vi "UHR-Fleezers Control (host) -TL FB Corrected Ronen semipassive - stepping.vi"(0 "Tab Control":T5(tab)=enum."Trap Control (RF)") -> ()   [LabVIEW 2013] (continued)
                    n948 = Wait (ms)(milliseconds to wait=u32 500) -> ()  [unwired: 1 out]
                  }
                  frame #4 {
                    n949 = call "Write to pump.vi"("string"="start", "VISA resource name"=w1515) -> ()  [unwired: 1 out]
                  }
                }
              }
            }
          }
          frame Enabled {
            n950 = call "hamilton_controller.vi"("Open?"=w1517, "valve"=enum16{"A", "B", "C", "D", "ALL"}."A", "action"=T21."MOVE VALVE") -> ()  [unwired: 8 in, 1 out]
          }
        }
      }
      event "Inject Valve B": Value Change {
        n951 = event-data() -> ()  [unwired: 7 out]
        n952 = disable-structure shown="Enabled" {
          disable-tunnel: "Inject Valve B" -> [w1521 w1541]
          frame Disabled {
            n953 = local read "Pump write delay (ms)"() -> (w1523:dbl)
            n954 = flat-sequence {
              tunnel: w1522 -> [w1536]
              tunnel: w1523 -> [w1532]
              tunnel: w1521 -> [_]
              tunnel: w1523 -> [w1538]
              tunnel: w1522 -> [w1539]
              frame #0 {
                n955 = local read "All Pump Parameters"() -> (w1531:T6)
                n956 = Multiply(x=60.0, y="Flush Center Ch Rate (ul/m)") -> (x*y=w1528:dbl)
                n957 = Unbundle By Name(w1531) -> ("Pump 2"=w1537:T33)
                n958 = call "Set pump parameters.vi"("Pump write delay (ms)"=w1532, "Volume (uL)"="Flush Center Ch Volume (uL)", "Rate (uL/h)"=w1528, "Units"=3.0, "Pump #"=2.0, "Pump Parameters In"=w1537, "VISA resource name"=w1536) -> ("Pump Parameters Out"=w1530:T33)  [unwired: 3 in]
                n959 = Bundle By Name(cluster=w1531, "Pump 2"=w1530) -> (w1529:T6)
                n960 = local write "All Pump Parameters"(w1529) -> ()
                n961 = Add(x="Flush Center Ch Volume (uL)", y="Total Volume\nFlushed (uL)") -> (x+y=w1525:dbl)
                n962 = local write "Total Volume\nFlushed (uL)"(w1525) -> ()
              }
              frame #1 {
                n963 = Wait (ms)(milliseconds to wait=w1538) -> ()  [unwired: 1 out]
              }
              frame #2 {
                n964 = call "Write to pump.vi"("string"="start", "VISA resource name"=w1539) -> ()  [unwired: 1 out]
              }
            }
            n965 = local read "Chemyx Syringe Pump Serial Port"() -> (w1522:refnum<visa-resource-name>)
          }
          frame Enabled {
            n966 = call "hamilton_controller.vi"("Open?"=w1541, "valve"=enum16{"A", "B", "C", "D", "ALL"}."B", "action"=T21."MOVE VALVE") -> ()  [unwired: 8 in, 1 out]
          }
        }
      }
      event "Inject Bottom": Value Change {
        n967 = event-data() -> ()  [unwired: 7 out]
        n968 = call "hamilton_controller.vi"("Open?"="Inject Bottom", "valve"=enum16{"A", "B", "C", "D", "ALL"}."C", "action"=T21."MOVE VALVE") -> ()  [unwired: 8 in, 1 out]
      }
      event "Shunt:": Value Change {
        n969 = event-data() -> ()  [unwired: 7 out]
        n970 = call "hamilton_controller.vi"("Open?"="Shunt:", "valve"=enum16{"A", "B", "C", "D", "ALL"}."D", "action"=T21."MOVE VALVE") -> ()  [unwired: 8 in, 1 out]
      }
      event "Flip Green Filter": Value Change {
        n971 = event-data() -> ()  [unwired: 7 out]
        n972 = local write "Flip Green Filter"("Flip Green Filter") -> ()
        n973 = flat-sequence {
          tunnel: w1557 -> [w1562]
          tunnel: w1556 -> [w1561]
          tunnel: [w1559] -> w1554
          tunnel: [w1558] -> w1553
          tunnel: [w1564] -> w1552
          tunnel: w1554 -> [w1564]
          tunnel: [w1563] -> w1551
          tunnel: w1553 -> [w1563]
          tunnel: w1552 -> [w1568]
          tunnel: w1551 -> [w1567]
          tunnel: [w1566] -> w1555
          frame #0 {
            n974 = xnode "Read/Write Control"("FPGA VI Reference In"=w1562, "error in"=w1561, "Green Filter Flipper"=TRUE) -> ("FPGA VI Reference Out"=w1559:T20, "error out"=w1558:errorcluster)
          }
          frame #1 {
            n975 = Wait (ms)(milliseconds to wait=u32 100) -> ()  [unwired: 1 out]
          }
          frame #2 {
            n976 = xnode "Read/Write Control"("FPGA VI Reference In"=w1568, "error in"=w1567, "Green Filter Flipper"=FALSE) -> ("error out"=w1566:errorcluster)  [unwired: 1 out]
          }
        }
      }
      event "Pump 1 contents", "Pump 3 contents": Value Change {
        n977 = event-data() -> ()  [unwired: 7 out]
        n978 = local read "Pump 1 contents"() -> (→"Pump 1 cont disp":string)
        n979 = local read "Pump 3 contents"() -> (→"Pump 3 cont disp":string)
      }
      event "Reset Trap Pos. FB": Value Change {
        n980 = event-data() -> ()  [unwired: 7 out]
        n981 = xnode "Read/Write Control"("FPGA VI Reference In"=w1574, "error in"=w1573, "Trap Pos. FB Reset"="Reset Trap Pos. FB") -> ()  [unwired: 2 out]
      }
      event "Trap Pos. FB ON": Value Change {
        n982 = event-data() -> ()  [unwired: 7 out]
        n983 = xnode "Read/Write Control"("FPGA VI Reference In"=w1589, "error in"=w1588) -> ("FPGA VI Reference Out"=w1586:T20, "BD1 Frequency Out 1"=w1583:u64)  [unwired: 1 out]
        n984 = To Double Precision Float(number=w1583) -> (double precision float=w1582:dbl)
        n985 = Multiply(x=49125000.0, y=6.0) -> (x*y=w1581:dbl)
        n986 = Multiply(x=w1582, y=w1581) -> (x*y=w1579:dbl)
        n987 = Scale By Power Of 2(n=-48, x=w1579) -> (x*2^n=w1578:dbl)
        n988 = Divide(x=w1578, y=1000000.0) -> (x/y=w1575:dbl)
        n989 = flat-sequence {
          tunnel: [w1592] -> w1587
          tunnel: w1586 -> [w1593]
          tunnel: w1583 -> [w1591]
          tunnel: "Trap Pos. FB ON" -> [w1590]
          tunnel: "Trap Pos. FB ON" -> [w1599]
          tunnel: w1587 -> [w1598]
          tunnel: "Trap Pos. FB ON" -> [w1601]
          tunnel: w1575 -> [w1600]
          frame #0 {
            n990 = case shown="False" w1590 {
              tunnel: w1593 -> [w1596 w1597]
              tunnel: [w1595 w1597] -> w1592
              tunnel: w1591 -> [w1594 _]
              frame False {
                n991 = xnode "Read/Write Control"("FPGA VI Reference In"=w1596, "BD 1 Frequency 1"=w1594) -> ("FPGA VI Reference Out"=w1595:T20)  [unwired: 1 in, 1 out]
              }
              frame True {
              }
            }
          }
          frame #1 {
            n992 = xnode "Read/Write Control"("FPGA VI Reference In"=w1598, "Force feedback"=w1599) -> ()  [unwired: 1 in, 2 out]
          }
          frame #2 {
            n993 = case shown="False" w1601 {
              tunnel: w1600 -> [w1603 _]
              frame False {
                n994 = Subtract(x=90.0, y=w1603) -> (x-y=w1602:dbl)
                n995 = property on="Trap Delta (MHz)" class="DigNum (strict)"("Val(Sgnl)"=w1602) -> ()  [unwired: 2 in, 2 out]
              }
              frame True {
              }
            }
          }
        }
      }
      event "Diff. FB.", "Trap Pos. FB Gains", "Trap Pos. FB Mult Factor", "Trap Pos. FB Offset Factor", "Trap Pos FB Negate Action", "Trap Pos FB Monitor\nT1 or T2", "Negate Diff?": Value Change {
        n996 = event-data() -> ()  [unwired: 7 out]
        n997 = xnode "Read/Write Control"("FPGA VI Reference In"=w1615, "error in"=w1614, "Trap Pos. FB Range"="Trap Pos. FB Range", "Trap Pos. FB Gains"="Trap Pos. FB Gains", "Trap Pos. FB Mult Factor"="Trap Pos. FB Mult Factor", "Trap Pos. FB Offset Factor"="Trap Pos. FB Offset Factor", "Trap Pos FB Negate Action"="Trap Pos FB Negate Action", "Trap Pos FB Monitor T1 or T2"="Trap Pos FB Monitor\nT1 or T2", "AI1 X Scale"="Trap Pos. AI1 X Pre-scale", "Negate Diff?"="Negate Diff?", "Diff FB Measurement?"="Diff. FB.") -> ()  [unwired: 2 out]
      }
      event "Trap Pos FB SP": Value Change {
        n998 = event-data() -> ()  [unwired: 7 out]
        n999 = xnode "Read/Write Control"("FPGA VI Reference In"=w1618, "error in"=w1617, "Trap Pos. FB SP"="Trap Pos FB SP") -> ()  [unwired: 2 out]
      }
      event "Simulate stepping": Value Change {
        n1000 = event-data() -> ()  [unwired: 7 out]
        n1001 = flat-sequence {
          tunnel: w1620 -> [w1623]
          tunnel: [w1622] -> _
          tunnel: w1619 -> [w1621]
          frame #0 {
            n1002 = while {
              tunnel: w1623 -> [w1651]
              tunnel: [w1650] -> w1622 mode=indexing
              tunnel: w1621 -> [w1649]
              i -> [w1635]
              stop <- w1632 stop-if-true
              w1625 = 1000.0
              n1003 = Divide(x="Backtrack probability", y=100) -> (x/y=w1659:dbl)
              n1004 = Random Number (0-1)() -> (number: 0 to 1=w1660:dbl)
              n1005 = Greater?(x=w1660, y=w1659) -> (0:w1658:bool)
              n1006 = Select(t=1, s=w1658, f=-1) -> (s? t:f=w1655:i32)
              n1007 = local read "BD 1 Frequency 2 (MHz)"() -> (w1630:dbl)
              n1008 = Multiply(x=w1655, y="Step size (nm)") -> (x*y=w1653:dbl)
              "Step taken" <- w1653
              n1009 = Divide(x=w1653, y=168.33) -> (x/y=w1628:dbl)
              n1010 = local read "BD 1 Frequency 1 (MHz)"() -> (w1629:dbl)
              n1011 = local read "X RF Frequency Limits (MHz)"() -> (w1648:T17)
              n1012 = local read "Y RF Frequency Limits (MHz)"() -> (w1647:T17)
              n1013 = Subtract(x=w1629, y=w1628) -> (x-y=w1627:dbl)
              n1014 = local write "BD 1 Frequency 1 (MHz)"(w1627) -> ()
              n1015 = local read "BD 2 Frequency 1 (MHz)"() -> (w1645:dbl)
              n1016 = local read "BD 2 Frequency 2 (MHz)"() -> (w1646:dbl)
              n1017 = call "set RF board frequency - interlace.vi"("Board 2 Frequency Limits"=w1647, "Board 1 Frequency Limits"=w1648, "error in"=w1651, "FPGA VI Reference In"=w1649, "Board 2 Frequency 2 (MHz)"=w1646, "Board 2 Frequency 1 (MHz)"=w1645, "Board 1 Frequency 2 (MHz)"=w1630, "Board 1 Frequency 1  (MHz)"=w1627) -> ("error out"=w1650:errorcluster)  [unwired: 2 in, 1 out]
              n1018 = Subtract(x=w1630, y=w1627) -> (x-y=w1644:dbl)
              n1019 = Subtract(x=w1646, y=w1645) -> (x-y=w1643:dbl)
              n1020 = Square(x=w1643) -> (x^2=w1641:dbl)
              n1021 = Square(x=w1644) -> (x^2=w1642:dbl)
              n1022 = Add(x=w1642, y=w1641) -> (x+y=w1640:dbl)
              n1023 = Square Root(x=w1640) -> (sqrt(x)=w1631:dbl)
              n1024 = local write "Trap Delta (MHz)"(w1631) -> ()
              n1025 = property on="Initial delta (MHz)" class="DigNum (strict)"("Val(Sgnl)"=w1631) -> ()  [unwired: 2 in, 2 out]
              n1026 = Multiply(x="Mean dwell time (s)", y=w1625) -> (x*y=w1637:dbl)
              n1027 = case shown="\"Gamma2\"" "Distribution" {
                tunnel: w1637 -> [w1664 w1668 w1671]
                tunnel: [w1664 w1665 w1672] -> w1626
                frame "uniform", Default {
                }
                frame "Exponential" {
                  n1028 = call-poly <vilib>:"Continuous Random.vi"("b"=w1668, "samples"=1) -> ("exp random data"=w1666:dbl[])  [unwired: 8 in, 1 out]
                  n1029 = Index Array(array=w1666) -> (element=w1665:dbl)  [unwired: 1 in]
                }
                frame "Gamma2" {
                  w1669 = 2.0
                  # "Note: the shape and scale\nparameters of the gamma\nare inverted because LabView..."
                  n1030 = Divide(x=w1671, y=w1669) -> (x/y=w1670:dbl)
                  n1031 = call-poly <vilib>:"Continuous Random.vi"("c"=w1670, "b"=w1669, "samples"=1) -> ("gamma random numbers"=w1673:dbl[])  [unwired: 7 in, 1 out]
                  n1032 = Index Array(array=w1673) -> (element=w1672:dbl)  [unwired: 1 in]
                }
              }
              n1033 = Divide(x=w1626, y=w1625) -> (x/y=→"Step duration":dbl)
              n1034 = To Unsigned Long Integer(number=w1626) -> (unsigned 32bit integer=w1638:u32)
              n1035 = Add(x=w1635, y=1) -> (x+y=w1634:i32)
              n1036 = Wait (ms)(milliseconds to wait=w1638) -> ()  [unwired: 1 out]
              n1037 = Equal?(x=w1634, y="Number of steps") -> (x = y?=w1632:bool)
            }
          }
          frame #1 {
            n1038 = local write "Simulate stepping"(FALSE) -> ()
          }
        }
      }
      event "Set SP to Reading": Value Change {
        n1039 = event-data() -> ()  [unwired: 7 out]
        n1040 = local read "Trap Pos FB Monitor\nT1 or T2"() -> (w1683:bool)
        n1041 = local read "Trap X AI1 (DMA)"() -> (w1686:T13)
        n1042 = local read "Trap X (AI1)"() -> (w1689:T1)
        n1043 = Unbundle By Name(w1689) -> ("Trap 1"=w1688:fxp<+/-,16,1>, "Trap 2"=w1687:fxp<+/-,16,1>)
        n1044 = Unbundle By Name(w1686) -> ("Set 1"=w1685:fxp<+/-,16,1>, "Set 2"=w1684:fxp<+/-,16,1>)
        n1045 = Select(t=w1688, s=w1683, f=w1687) -> (s? t:f=w1682:fxp<+/-,16,1>)
        n1046 = Select(t=w1685, s=w1683, f=w1684) -> (s? t:f=w1681:fxp<+/-,16,1>)
        n1047 = Not(x="Set SP Using...") -> (.not. x?=w1676:bool)
        n1048 = Select(t=w1682, s=w1676, f=w1681) -> (s? t:f=w1677:fxp<+/-,16,1>)
        n1049 = xnode "Read/Write Control"("FPGA VI Reference In"=w1679, "error in"=w1678, "Trap Pos. FB SP"=w1677) -> ()  [unwired: 2 out]
        n1050 = local write "Trap Pos FB SP"(w1677) -> ()
      }
      event "Trap Pos. FB Out Scale 2^n": Value Change {
        n1051 = event-data() -> ()  [unwired: 7 out]
        n1052 = Scale By Power Of 2(n="Trap Pos. FB Out Scale 2^n", x=ext 1.0) -> (x*2^n=w1691:ext)
        n1053 = property on="Trap Pos. FB Mult Factor" class="DigNum (strict)"("Val(Sgnl)"=w1691) -> ()  [unwired: 2 in, 2 out]
      }
      event "Trap Pos FB Int Count": Value Change {
        n1054 = event-data() -> ()  [unwired: 7 out]
        n1055 = xnode "Read/Write Control"("FPGA VI Reference In"=w1696, "error in"=w1695, "Trap Pos FB Int Count"="Trap Pos FB Int Count") -> ()  [unwired: 2 out]
      }
      event "Target Force (pN)", "Setpoint offset\nCorrection values": Value Change {
        n1056 = event-data() -> ()  [unwired: 7 out]
        n1057 = local read "B factor"() -> (w1729:dbl)
        n1058 = To Fixed-Point(number=w1729) -> (fixed-point=w1728:fxp<+/-,16,16>)  [unwired: 1 in]
        n1059 = xnode "Read/Write Control"("FPGA VI Reference In"=w1730, "B factor"=w1728) -> ("BD1 Frequency Out 1"=w1719:u64)  [unwired: 1 in, 2 out]
        n1060 = local read "BD 1 Frequency 2 (MHz)"() -> (w1718:dbl)
        n1061 = local read "Target Force (pN)"() -> (w1704:dbl)
        n1062 = To Double Precision Float(number=w1719) -> (double precision float=w1725:dbl)
        n1063 = Multiply(x=49125000.0, y=6.0) -> (x*y=w1724:dbl)
        n1064 = Multiply(x=w1725, y=w1724) -> (x*y=w1722:dbl)
        n1065 = Scale By Power Of 2(n=-48, x=w1722) -> (x*2^n=w1721:dbl)
        n1066 = Divide(x=w1721, y=1000000.0) -> (x/y=w1717:dbl)
        n1067 = Subtract(x=w1718, y=w1717) -> (x-y=w1716:dbl)
        n1068 = local read "T1 kappa_x (pN/nm)"() -> (w1705:dbl)
        n1069 = local read "T1 alpha_x (nm/V)"() -> (w1706:dbl)
        n1070 = local read "Negate offset difference"() -> (w1707:bool)
        n1071 = local read "Offset file step size"() -> (w1715:dbl)
        n1072 = Multiply(x=w1704, y=2.0) -> (x*y=w1702:dbl)
        n1073 = local read "Setpoint offset\nCorrection values"() -> (w1712:dbl[])
        n1074 = Divide(x=w1716, y=w1715) -> (x/y=w1714:dbl)
        n1075 = Select(t=-1, s=w1707, f=1) -> (s? t:f=w1708:i32)
        n1076 = To Long Integer(number=w1714) -> (32bit integer=w1713:i32)
        n1077 = Multiply(x=w1706, y=w1705) -> (x*y=w1701:dbl)
        n1078 = Divide(x=w1702, y=w1701) -> (x/y=w1700:dbl)
        n1079 = Index Array(array=w1712, index=w1713) -> (element=w1711:dbl)
        n1080 = Multiply(x=w1708, y=w1711) -> (x*y=w1699:dbl)
        n1081 = Add(x=w1700, y=w1699) -> (x+y=w1698:dbl)
        n1082 = To Fixed-Point(number=w1698) -> (fixed-point=w1697:fxp<+/-,16,1>)  [unwired: 1 in]
        n1083 = property on="Trap Pos FB SP" class="DigNum (strict)"("Val(Sgnl)"=w1697) -> ()  [unwired: 2 in, 2 out]
      }
      event "Read setpoint correction\nfile": Value Change {
        n1084 = event-data() -> ()  [unwired: 7 out]
        n1085 = local write "Read setpoint correction\nfile"(FALSE) -> ()
        n1086 = Open/Create/Replace File(file path (use dialog)="Setpoint correction\noffset file", operation (0:open)=T24."open", access (0:read/write)=enum16{"read/write", "read-only", "write-only"}."read-only") -> (refnum out=w1755:refnum<file>)  [unwired: 1 in, 4 out]
        n1087 = Deny Access(7:w1755) -> (3:w1753:refnum<file>)  [unwired: 1 in, 2 out]
        n1088 = Read from Binary File(5:0.0, 9:T30."big-endian, network order" ("byte order (0:big-endian, network order)"), 10:-1 ("count (1)"), 11:w1753) -> (2:w1746:dbl[], 3:w1752:refnum<file>)  [unwired: 1 in, 3 out]
        n1089 = Close File(refnum=w1752) -> ()  [unwired: 1 in, 2 out]
        n1090 = Index Array(array=w1746, index=0) -> (element=w1742:dbl)
        n1091 = local write "Offset file step size"(w1742) -> ()
        n1092 = Array Subset(array=w1746, index=3) -> (w1745:dbl[])  [unwired: 1 in]
        n1093 = local read "T1 kappa_x (pN/nm)"() -> (w1740:dbl)
        n1094 = local read "T1 alpha_x (nm/V)"() -> (w1741:dbl)
        n1095 = local read "T2 alpha_x (nm/V)"() -> (w1739:dbl)
        n1096 = local read "T2 kappa_x (pN/nm)"() -> (w1738:dbl)
        n1097 = Decimate 1D Array(w1745) -> (w1733:dbl[], w1734:dbl[])  [unwired: 1 out]
        n1098 = local read "Offset Values"() -> (w1744:T14)
        n1099 = Multiply(x=w1741, y=w1740) -> (x*y=w1736:dbl)
        n1100 = Multiply(x=w1739, y=w1738) -> (x*y=w1737:dbl)
        n1101 = Bundle By Name(cluster=w1744, "Trap 1X offset"=w1733, "Trap 2X offset"=w1734) -> (w1743:T14)
        n1102 = Divide(x=w1737, y=w1736) -> (x/y=w1735:dbl)
        n1103 = property on="B factor" class="DigNum (strict)"("Val(Sgnl)"=w1735) -> ()  [unwired: 2 in, 2 out]
        n1104 = Multiply(x=w1734, y=w1735) -> (x*y=w1732:dbl[])
        n1105 = local write "Offset Values"(w1743) -> ()
        n1106 = Subtract(x=w1733, y=w1732) -> (x-y=w1731:dbl[])
        n1107 = property on="Setpoint offset\nCorrection values" class="Arr (strict)"("Val(Sgnl)"=w1731) -> ()  [unwired: 2 in, 2 out]
      }
      event "MCL Tracking": Value Change {
        n1108 = event-data() -> ()  [unwired: 7 out]
        n1109 = case shown="True" "MCL Tracking" {
          frame False {
            n1110 = local read "Current MCL (V)"() -> (w1760:dbl)
            n1111 = local write "AO2"(w1760) -> ()
          }
          frame True {
            n1112 = local read "BD 1 Frequency 1 (MHz)"() -> (→"Zero T1 position":dbl)
            n1113 = local read "AO2"() -> (→"Zero MCL x position":dbl)
          }
        }
      }
    }
    "error out 2" <- w754
    n1114 = node-c288() -> ()  [unwired: 1 in, 1 out]
  }
  n1115 = timed-loop "Run Scripts, including: stage motion" {
    timing: w89 -> [_]
    timing-out: [_] -> w88
    tunnel: w44 -> [_]
    stop <- w1764 stop-if-true
    n1116 = node-c288() -> ()  [unwired: 1 in, 1 out]
    n1117 = event shown="[2] \"Cal/Data Acq. Spot\": Value Change" {
      selector: _ -> [_ _ _ _ _ _ _ _ _ _ _ _]
      dyn-events: _ -> [_ _ _ _ _ _ _ _ _ _ _ _]
      timeout: 50 -> [_ _ _ _ _ _ _ _ _ _ _ _]
      tunnel: ["Move Cap. 1 (DNA Top)" _ "Cal/Data Acq. Spot" "Dump Beads" "Dip for Protein" _ "Got ADig bead" "Got DNA bead" "Take Stepping Data" _ "Take Detection Laser\nImage" _] -> _
      tunnel: [_ _ _ _ _ _ _ _ _ _ _ w1972] -> w1764
      event "Move Cap. 1 (DNA Top)": Value Change {
        n1118 = event-data() -> ()  [unwired: 1 in, 5 out]
        n1119 = local write "Move Cap. 1 (DNA Top)"(FALSE ("Move Cap. 1 (DNA Right)")) -> ()
        n1120 = flat-sequence {
          tunnel: "Cap 1 Samp Flow ON" -> [w1770]
          frame #0 {
            n1121 = local write "Stage Moving"(FALSE ("Stage Moving")) -> ()
            n1122 = case "stop flow" shown="True" w1770 {
              frame False {
              }
              frame True {
                n1123 = call "hamilton_controller.vi"("Open?"=FALSE, "valve"=enum16{"A", "B", "C", "D", "ALL"}."C", "action"=T21."MOVE VALVE") -> ()  [unwired: 8 in, 1 out]
              }
            }
            n1124 = case shown="True" TRUE {
              tunnel: "Cap 1 T ON" -> [w1779 w1780]
              frame False {
                n1125 = property on="Trap 1 (ON/OFF)" class="Bool (strict)"("Val(Sgnl)"=w1779) -> ()  [unwired: 2 in, 2 out]
              }
              frame True {
                n1126 = property on="Trap 2 (ON/OFF)" class="Bool (strict)"("Val(Sgnl)"=w1780) -> ()  [unwired: 2 in, 2 out]
              }
            }
            n1127 = call <vilib>:"Beep.vi"() -> ()  [unwired: 3 in, 9 out]
            n1128 = case shown="True" "Cap 1 Flow ON" {
              frame False {
              }
              frame True {
                n1129 = property on="Main:" class="Bool (strict)"("Val(Sgnl)"=TRUE ("Value (Signaling)")) -> ()  [unwired: 2 in, 2 out]
              }
            }
          }
        }
      }
      event Timeout {
        n1130 = event-data() -> ()  [unwired: 1 in, 2 out]
      }
      event "Cal/Data Acq. Spot": Value Change {
        # "wait for calibration file\nto be written"
        # "signal save cal true\nthis tells the data \nacquisition loop to\nstart sending the data\nto a calibration file"
        # "separate traps to\nthe desired trap delta"
        # "move stage to data acquisition spot"
        # "CHANGE FISH FOR TETHER BACK\nTO TRUE VALUE HERE."
        n1131 = event-data() -> ()  [unwired: 1 in, 5 out]
        n1132 = local write "Cal/Data Acq. Spot"(FALSE ("Cal/Data Acq. Spot")) -> ()
        n1133 = flat-sequence {
          tunnel: ["Cal @ (MHz)"] -> w1781
          tunnel: w1781 -> [w1791]
          tunnel: w1781 -> [w1812]
          frame #0 {
            n1134 = property on="Trap Delta (MHz)" class="DigNum (strict)"("Val(Sgnl)"="Cal @ (MHz)") -> ()  [unwired: 2 in, 2 out]
            n1135 = call <vilib>:"Beep.vi"() -> ()  [unwired: 3 in, 9 out]
          }
          frame #1 {
            n1136 = Wait (ms)(milliseconds to wait=u32 100) -> ()  [unwired: 1 out]
          }
          frame #2 {
            n1137 = property on="Save Calibration" class="Bool (strict)"("Val(Sgnl)"=TRUE ("Value (Signaling)")) -> ()  [unwired: 2 in, 2 out]
          }
          frame #3 {
            n1138 = Wait (ms)(milliseconds to wait=u32 4000) -> ()  [unwired: 1 out]
          }
          frame #4 {
            n1139 = while {
              stop <- w1788 stop-if-true
              n1140 = local read "Saving..."() -> (w1789:bool)
              n1141 = Wait (ms)(milliseconds to wait=u32 100) -> ()  [unwired: 1 out]
              n1142 = Not(x=w1789) -> (.not. x?=w1788:bool)
            }
          }
          frame #5 {
            n1143 = case shown="True" "W/ Offset 1" {
              tunnel: w1791 -> [_ w1793]
              frame False {
              }
              frame True {
                n1144 = stacked-sequence {
                  tunnel: w1793 -> [_ _ _ _ _ _ _ w1810]
                  frame #0 {
                    n1145 = Replace Array Subset(array=u32[] [0] ("Index Values"), new element="Offset 1 Set", index=0) -> (w1794:u32[])
                    n1146 = property on="Saved AOD Raster Scan Parameter Sets" class="Arr (strict)"("Index Values"=w1794) -> ()  [unwired: 2 in, 2 out]
                    n1147 = property on="Trap Delta (MHz)" class="DigNum (strict)"("Val(Sgnl)"="Offset 1 Start (MHz)") -> ()  [unwired: 2 in, 2 out]
                  }
                  frame #1 {
                    n1148 = Wait (ms)(milliseconds to wait=u32 200) -> ()  [unwired: 1 out]
                  }
                  frame #2 {
                    n1149 = property on="Load parameters" class="Bool (strict)"("Val(Sgnl)"=TRUE ("Value (Signaling)")) -> ()  [unwired: 2 in, 2 out]
                  }
                  frame #3 {
                    n1150 = Wait (ms)(milliseconds to wait=u32 200) -> ()  [unwired: 1 out]
                  }
                  frame #4 {
                    n1151 = property on="Trap Raster Scan" class="Bool (strict)"("Val(Sgnl)"=TRUE ("Value (Signaling)")) -> ()  [unwired: 2 in, 2 out]
                  }
                  frame #5 {
                    n1152 = Wait (ms)(milliseconds to wait=u32 2000) -> ()  [unwired: 1 out]
                  }
                  frame #6 {
                    n1153 = while {
                      stop <- w1807 stop-if-true
                      n1154 = local read "Raster Scanning..."() -> (w1809:bool)
                      n1155 = local read "Saving..."() -> (w1805:bool)
                      n1156 = Wait (ms)(milliseconds to wait=u32 100) -> ()  [unwired: 1 out]
                      n1157 = Not(x=w1805) -> (.not. x?=w1804:bool)
                      n1158 = Not(x=w1809) -> (.not. x?=w1806:bool)
                      n1159 = And(x=w1806, y=w1804) -> (x .and. y?=w1807:bool)
                    }
                  }
                  frame #7 {
                    n1160 = property on="Trap Delta (MHz)" class="DigNum (strict)"("Val(Sgnl)"=w1810) -> ()  [unwired: 2 in, 2 out]
                  }
                }
              }
            }
          }
          frame #6 {
            n1161 = local read "Save ave N"() -> (w1811:dbl)
            n1162 = case shown="True" "W/ Offset 2" {
              tunnel: w1812 -> [_ w1818]
              tunnel: w1811 -> [_ w1817]
              frame False {
                n1163 = Multiply(x="Cal read wait (s)", y=u32 1000 ("milliseconds to wait")) -> (x*y=w1815:u32)
                n1164 = Wait (ms)(milliseconds to wait=w1815) -> ()  [unwired: 1 out]
              }
              frame True {
                n1165 = stacked-sequence {
                  tunnel: w1818 -> [_ _ _ _ _ _ _ _ _ w1839 _ _]
                  tunnel: w1817 -> [_ _ _ _ _ _ _ _ _ w1837 _ _]
                  frame #0 {
                    n1166 = property on="Save ave N" class="DigNum (strict)"("Val(Sgnl)"=1.0 ("Value (Signaling)")) -> ()  [unwired: 2 in, 2 out]
                  }
                  frame #1 {
                    n1167 = Wait (ms)(milliseconds to wait=u32 500) -> ()  [unwired: 1 out]
                  }
                  frame #2 {
                    n1168 = property on="Trap Delta (MHz)" class="DigNum (strict)"("Val(Sgnl)"="Offset 2 Start (MHz)") -> ()  [unwired: 2 in, 2 out]
                    n1169 = Replace Array Subset(array=u32[] [0] ("Index Values"), new element="Offset 2 Set", index=0) -> (w1823:u32[])
                    n1170 = property on="Saved AOD Raster Scan Parameter Sets" class="Arr (strict)"("Index Values"=w1823) -> ()  [unwired: 2 in, 2 out]
                  }
                  frame #3 {
                    n1171 = Wait (ms)(milliseconds to wait=u32 500) -> ()  [unwired: 1 out]
                  }
                  frame #4 {
                    n1172 = property on="Load parameters" class="Bool (strict)"("Val(Sgnl)"=TRUE ("Value (Signaling)")) -> ()  [unwired: 2 in, 2 out]
                  }
                  frame #5 {
                    n1173 = Wait (ms)(milliseconds to wait=u32 500) -> ()  [unwired: 1 out]
                  }
                  frame #6 {
                    n1174 = property on="Trap Raster Scan" class="Bool (strict)"("Val(Sgnl)"=TRUE ("Value (Signaling)")) -> ()  [unwired: 2 in, 2 out]
                  }
                  frame #7 {
                    n1175 = Wait (ms)(milliseconds to wait=u32 2000) -> ()  [unwired: 1 out]
                  }
                  frame #8 {
                    n1176 = while {
                      stop <- w1832 stop-if-true
                      n1177 = local read "Raster Scanning..."() -> (w1835:bool)
                      n1178 = local read "Saving..."() -> (w1833:bool)
                      n1179 = Wait (ms)(milliseconds to wait=u32 100) -> ()  [unwired: 1 out]
                      n1180 = Not(x=w1833) -> (.not. x?=w1831:bool)
                      n1181 = Not(x=w1835) -> (.not. x?=w1834:bool)
                      n1182 = And(x=w1834, y=w1831) -> (x .and. y?=w1832:bool)
                    }
                  }
                  frame #9 {
                    n1183 = property on="Trap Delta (MHz)" class="DigNum (strict)"("Val(Sgnl)"=w1839) -> ()  [unwired: 2 in, 2 out]
                    n1184 = property on="Saved AOD Raster Scan Parameter Sets" class="Arr (strict)"("Index Values"=u32[] [0]) -> ()  [unwired: 2 in, 2 out]
                    n1185 = property on="Save ave N" class="DigNum (strict)"("Val(Sgnl)"=w1837) -> ()  [unwired: 2 in, 2 out]
                  }
                  frame #10 {
                    n1186 = Wait (ms)(milliseconds to wait=u32 500) -> ()  [unwired: 1 out]
                  }
                  frame #11 {
                    n1187 = property on="Load parameters" class="Bool (strict)"("Val(Sgnl)"=TRUE ("Value (Signaling)")) -> ()  [unwired: 2 in, 2 out]
                  }
                }
              }
            }
          }
          frame #7 {
            n1188 = property on="Read Cal" class="Bool (strict)"("Val(Sgnl)"=TRUE ("Value (Signaling)")) -> ()  [unwired: 2 in, 2 out]
          }
          frame #8 {
            n1189 = Wait (ms)(milliseconds to wait=u32 500) -> ()  [unwired: 1 out]
          }
          frame #9 {
            n1190 = property on="Fish for Tether" class="Bool (strict)"("Val(Sgnl)"=FALSE ("Value (Signaling)")) -> ()  [unwired: 2 in, 2 out]
          }
        }
      }
      event "Dump Beads": Value Change {
        # "SCRIPT TO REMOVE BOTH BEADS FROM THE TRAPS. TURNS ON LIGHT WHICH INDICATES THAT STAGE IS MOVING. THEN STOPS SAVING DATA. \nSETS Sample Channel Flow TO TRUE. STOPS INTERLACING GREEN FLUORESCENCE. TURNS OFF Tether INDICATOR BECAUSE WE ARE THROWING IT\nAWAY. SHUTS OFF TRAP POSITION FEEDBACK."
        n1191 = event-data() -> ()  [unwired: 1 in, 5 out]
        n1192 = flat-sequence {
          frame #0 {
            w1846 = FALSE ("Fl. Triggered...")
            w1847 = TRUE ("Stage Moving")
            n1193 = local read "Saving..."() -> (w1848:bool)
            n1194 = local write "Fl. Triggered..."(w1846) -> ()
            n1195 = local write "Stage Moving"(w1847) -> ()
            n1196 = local write "Tether"(w1846) -> ()
            n1197 = property on="Green Laser ON/Interlacing" class="Bool (strict)"("Val(Sgnl)"=w1846) -> ()  [unwired: 2 in, 2 out]
            n1198 = property on="Trap Pos. FB ON" class="Bool (strict)"("Val(Sgnl)"=w1846) -> ()  [unwired: 2 in, 2 out]
            n1199 = property on="Inject Bottom" class="Bool (strict)"("Val(Sgnl)"=w1847) -> ()  [unwired: 2 in, 2 out]
            n1200 = local write "Stop Saving"(w1848) -> ()
          }
          frame #1 {
            w1849 = FALSE ("Value (Signaling)")
            # "TURNS TRAPS OFF SO THAT\nBEADS REMAIN AT DUMP \nBEADS POSITION"
            n1201 = property on="Trap 1 (ON/OFF)" class="Bool (strict)"("Val(Sgnl)"=w1849) -> ()  [unwired: 2 in, 2 out]
            n1202 = property on="Trap 2 (ON/OFF)" class="Bool (strict)"("Val(Sgnl)"=w1849) -> ()  [unwired: 2 in, 2 out]
            n1203 = call <vilib>:"Beep.vi"() -> ()  [unwired: 3 in, 9 out]
          }
          frame #2 {
            n1204 = property on="Goto Bottom (F7)" class="Bool (strict)"("Val(Sgnl)"=TRUE ("Value (Signaling)")) -> ()  [unwired: 2 in, 2 out]
          }
          frame #3 {
            n1205 = Wait (ms)(milliseconds to wait=u32 8000) -> ()  [unwired: 1 out]
          }
          frame #4 {
            n1206 = property on="Trap Delta (MHz)" class="DigNum (strict)"("Val(Sgnl)"=20.0 ("Value (Signaling)")) -> ()  [unwired: 2 in, 2 out]
          }
          frame #5 {
            n1207 = property on="Trap 2 (ON/OFF)" class="Bool (strict)"("Val(Sgnl)"=TRUE ("Value (Signaling)")) -> ()  [unwired: 2 in, 2 out]
          }
          frame #6 {
            n1208 = property on="Inject Bottom" class="Bool (strict)"("Val(Sgnl)"=FALSE ("Value (Signaling)")) -> ()  [unwired: 2 in, 2 out]
          }
        }
      }
      event "Dip for Protein": Value Change {
        n1209 = event-data() -> ()  [unwired: 1 in, 5 out]
        n1210 = flat-sequence {
          frame #0 {
            n1211 = case shown="True" "Move Trap Before?" {
              frame False {
              }
              frame True {
                n1212 = property on="Trap Delta (MHz)" class="DigNum (strict)"("Val(Sgnl)"="Dip Trap Delta 1 (MHz)") -> ()  [unwired: 2 in, 2 out]
              }
            }
          }
          frame #1 {
            n1213 = Multiply(x="Duration (s)", y=1000.0) -> (x*y=w1858:dbl)
            n1214 = Wait (ms)(milliseconds to wait=w1858) -> ()  [unwired: 1 out]
          }
          frame #2 {
            n1215 = case shown="True" "Move Trap After?" {
              frame False {
              }
              frame True {
                n1216 = property on="Trap Delta (MHz)" class="DigNum (strict)"("Val(Sgnl)"="Dip Trap Delta 2 (MHz)") -> ()  [unwired: 2 in, 2 out]
              }
            }
          }
          frame #3 {
            n1217 = case shown="True" "Green ON After?" {
              frame False {
              }
              frame True {
                n1218 = property on="Green Laser ON/Interlacing" class="Bool (strict)"("Val(Sgnl)"=TRUE ("Value (Signaling)")) -> ()  [unwired: 2 in, 2 out]
              }
            }
          }
          frame #4 {
            n1219 = Wait (ms)(milliseconds to wait=u32 500) -> ()  [unwired: 1 out]
          }
          frame #5 {
            n1220 = case shown="True" "Save Data After?" {
              frame False {
              }
              frame True {
                n1221 = property on="Start Saving" class="Bool (strict)"("Val(Sgnl)"=TRUE ("Value (Signaling)")) -> ()  [unwired: 2 in, 2 out]
              }
            }
          }
        }
      }
      event "Profile": Value Change {
        n1222 = event-data() -> ()  [unwired: 1 in, 5 out]
        n1223 = flat-sequence {
          frame #0 {
            w1868 = 0.0 ("element")
            n1224 = Build Array(w1868, "Y change (mm)", w1868) -> ()  [unwired: 1 out]
          }
          frame #1 {
            # "stop saving"
            n1225 = local write "Stop Saving"(TRUE ("Stop Saving")) -> ()
            n1226 = local write "Stage Moving"(FALSE ("Stage Moving")) -> ()
          }
        }
      }
      event "Got ADig bead": Value Change {
        n1227 = event-data() -> ()  [unwired: 1 in, 5 out]
        n1228 = property on="Move Cap. 1 (DNA Top)" class="Bool (strict)"("Val(Sgnl)"=TRUE ("Value (Signaling)")) -> ()  [unwired: 2 in, 2 out]
        n1229 = property on="Inject Top:" class="Bool (strict)"("Val(Sgnl)"=FALSE ("Value (Signaling)")) -> ()  [unwired: 2 in, 2 out]
      }
      event "Got DNA bead": Value Change {
        n1230 = event-data() -> ()  [unwired: 1 in, 5 out]
        n1231 = property on="Cal/Data Acq. Spot" class="Bool (strict)"("Val(Sgnl)"=TRUE ("Value (Signaling)")) -> ()  [unwired: 2 in, 2 out]
        n1232 = property on="Main:" class="Bool (strict)"("Val(Sgnl)"=FALSE ("Value (Signaling)")) -> ()  [unwired: 2 in, 2 out]
      }
      event "Take Stepping Data": Value Change {
        n1233 = event-data() -> ()  [unwired: 1 in, 5 out]
        n1234 = local read "Save ave N"() -> (w1886:dbl)
        n1235 = flat-sequence {
          tunnel: w1886 -> [w1888]
          tunnel: [w1888] -> w1881
          tunnel: [w1890] -> w1882
          tunnel: w1881 -> [w1890]
          tunnel: [w1892] -> w1883
          tunnel: w1882 -> [w1892]
          tunnel: [w1895] -> w1884
          tunnel: w1883 -> [w1895]
          tunnel: [w1897] -> w1885
          tunnel: w1884 -> [w1897]
          tunnel: [w1899] -> w1879
          tunnel: w1885 -> [w1899]
          tunnel: w1879 -> [w1902]
          tunnel: [w1902] -> w1878
          tunnel: w1878 -> [w1903]
          tunnel: [w1903] -> w1880
          tunnel: w1880 -> [w1909]
          frame #0 {
            n1236 = property on="Save ave N" class="DigNum (strict)"("Val(Sgnl)"="Save ave factor") -> ()  [unwired: 2 in, 2 out]
          }
          frame #1 {
            n1237 = Wait (ms)(milliseconds to wait=u32 100) -> ()  [unwired: 1 out]
          }
          frame #2 {
            n1238 = local read "Offset 2 Start (MHz)"() -> (w1894:dbl)
            n1239 = property on="Saved AOD Raster Scan Parameter Sets" class="Arr (strict)"("Index Values"=u32[] [2]) -> ()  [unwired: 2 in, 2 out]
            n1240 = property on="Trap Delta (MHz)" class="DigNum (strict)"("Val(Sgnl)"=w1894) -> ()  [unwired: 2 in, 2 out]
          }
          frame #3 {
            n1241 = property on="Load parameters" class="Bool (strict)"("Val(Sgnl)"=TRUE ("Value (Signaling)")) -> ()  [unwired: 2 in, 2 out]
          }
          frame #4 {
            n1242 = Wait (ms)(milliseconds to wait=u32 100) -> ()  [unwired: 1 out]
          }
          frame #5 {
            n1243 = property on="Trap Raster Scan" class="Bool (strict)"("Val(Sgnl)"=TRUE ("Value (Signaling)")) -> ()  [unwired: 2 in, 2 out]
          }
          frame #6 {
            n1244 = Wait (ms)(milliseconds to wait=u32 1000) -> ()  [unwired: 1 out]
          }
          frame #7 {
            n1245 = while {
              stop <- w1906 stop-if-true
              n1246 = local read "Raster Scanning..."() -> (w1908:bool)
              n1247 = local read "Saving..."() -> (w1907:bool)
              n1248 = Not(x=w1907) -> (.not. x?=w1904:bool)
              n1249 = Not(x=w1908) -> (.not. x?=w1905:bool)
              n1250 = And(x=w1905, y=w1904) -> (x .and. y?=w1906:bool)
            }
          }
          frame #8 {
            n1251 = property on="Save ave N" class="DigNum (strict)"("Val(Sgnl)"=w1909) -> ()  [unwired: 2 in, 2 out]
          }
        }
      }
      event "Step Size (nm)": Value Change {
        n1252 = event-data() -> ()  [unwired: 1 in, 5 out]
        n1253 = flat-sequence {
          frame #0 {
            n1254 = property on="Saved AOD Raster Scan Parameter Sets" class="Arr (strict)"("Index Values"=u32[] [1]) -> ()  [unwired: 2 in, 2 out]
          }
          frame #1 {
            n1255 = Multiply(x="N Steps", y="Step Size (nm)") -> (x*y=w1911:dbl)
            n1256 = property on="Scan Speed AOD (nm/s) 2" class="DigNum (strict)"("Value"="Step Size (nm)") -> ()  [unwired: 2 in, 2 out]
            n1257 = property on="Step Size AOD (nm) 2" class="DigNum (strict)"("Value"="Step Size (nm)") -> ()  [unwired: 2 in, 2 out]
            n1258 = property on="Scan Range AOD (nm) 2" class="DigNum (strict)"("Value"=w1911) -> ()  [unwired: 2 in, 2 out]
          }
        }
      }
      event "Take Detection Laser\nImage": Value Change {
        n1259 = event-data() -> ()  [unwired: 1 in, 5 out]
        n1260 = flat-sequence {
          tunnel: [w1939] -> w1929
          tunnel: [w1938] -> w1922
          tunnel: [w1937] -> w1914
          tunnel: [w1942] -> w1930
          tunnel: w1929 -> [w1942]
          tunnel: [w1941] -> w1923
          tunnel: w1922 -> [w1941]
          tunnel: [w1940] -> w1915
          tunnel: w1914 -> [w1940]
          tunnel: [w1946] -> w1931
          tunnel: w1930 -> [w1946]
          tunnel: [w1945] -> w1924
          tunnel: w1923 -> [w1945]
          tunnel: [w1944] -> w1916
          tunnel: w1915 -> [w1944]
          tunnel: [w1952] -> w1932
          tunnel: w1931 -> [w1952]
          tunnel: [w1951] -> w1925
          tunnel: w1924 -> [w1951]
          tunnel: [w1950] -> w1917
          tunnel: w1916 -> [w1950]
          tunnel: [w1956] -> w1933
          tunnel: w1932 -> [w1956]
          tunnel: [w1955] -> w1926
          tunnel: w1925 -> [w1955]
          tunnel: [w1954] -> w1918
          tunnel: w1917 -> [w1954]
          tunnel: [w1960] -> w1934
          tunnel: w1933 -> [w1960]
          tunnel: [w1959] -> w1927
          tunnel: w1926 -> [w1959]
          tunnel: [w1958] -> w1919
          tunnel: w1918 -> [w1958]
          tunnel: [w1964] -> w1935
          tunnel: w1934 -> [w1964]
          tunnel: [w1963] -> w1928
          tunnel: w1927 -> [w1963]
          tunnel: [w1962] -> w1920
          tunnel: w1919 -> [w1962]
          tunnel: w1935 -> [w1970]
          tunnel: w1928 -> [w1969]
          tunnel: [w1967] -> w1921
          tunnel: w1920 -> [w1967]
          tunnel: w1921 -> [w1971]
          frame #0 {
            n1261 = local read "Green Laser ON/Interlacing"() -> (w1939:bool)
            n1262 = local read "Green laser mode"() -> (w1938:enum32{"Laser ON", "Laser OFF", "Interlace"})
            n1263 = local read "Green FB On/Off"() -> (w1937:bool)
          }
          frame #1 {
            n1264 = property on="Green FB On/Off" class="Bool (strict)"("Val(Sgnl)"=FALSE ("Value (Signaling)")) -> ()  [unwired: 2 in, 2 out]
          }
          frame #2 {
            n1265 = property on="Green Laser ON/Interlacing" class="Bool (strict)"("Val(Sgnl)"=TRUE ("Value (Signaling)")) -> ()  [unwired: 2 in, 2 out]
            n1266 = property on="Flip Green Filter" class="Bool (strict)"("Val(Sgnl)"=TRUE ("Value (Signaling)")) -> ()  [unwired: 2 in, 2 out]
            n1267 = property on="Green laser mode" class="RadioBtnsControl (strict)"("Val(Sgnl)"=enum32{"Laser ON", "Laser OFF", "Interlace"}."Laser ON" ("Value (Signaling)")) -> ()  [unwired: 2 in, 2 out]
          }
          frame #3 {
            n1268 = Wait (ms)(milliseconds to wait=u32 500) -> ()  [unwired: 1 out]
          }
          frame #4 {
            n1269 = property on="Confocal Image" class="Bool (strict)"("Val(Sgnl)"=TRUE ("Value (Signaling)")) -> ()  [unwired: 2 in, 2 out]
          }
          frame #5 {
            n1270 = Wait (ms)(milliseconds to wait=u32 2000) -> ()  [unwired: 1 out]
          }
          frame #6 {
            n1271 = while {
              stop <- w1965 stop-if-true
              n1272 = local read "Saving..."() -> (w1966:bool)
              n1273 = Not(x=w1966) -> (.not. x?=w1965:bool)
            }
          }
          frame #7 {
            n1274 = property on="Flip Green Filter" class="Bool (strict)"("Val(Sgnl)"=TRUE ("Value (Signaling)")) -> ()  [unwired: 2 in, 2 out]
            n1275 = property on="Green Laser ON/Interlacing" class="Bool (strict)"("Val(Sgnl)"=w1970) -> ()  [unwired: 2 in, 2 out]
            n1276 = property on="Green laser mode" class="RadioBtnsControl (strict)"("Val(Sgnl)"=w1969) -> ()  [unwired: 2 in, 2 out]
          }
          frame #8 {
            n1277 = property on="Green FB On/Off" class="Bool (strict)"("Val(Sgnl)"=w1971) -> ()  [unwired: 2 in, 2 out]
          }
        }
      }
      event "Stop All": Value Change {
        n1278 = event-data() -> ()  [unwired: 1 in, 5 out]
        n1279 = local read "Stop All"() -> (w1972:bool)
      }
    }
    n1280 = node-c288() -> ()  [unwired: 1 in, 1 out]
  }
  n1281 = node-c288() -> (w96:T25)  [unwired: 4 out]
  n1282 = timed-loop "Mouse control: trap position (AOM deflection), set confocal spot from image" {
    tunnel: [w1974] -> w54
    tunnel: w44 -> [w1973]
    timing: w96 -> [_]
    timing-out: [_] -> w95
    stop <- w1974 stop-if-true
    n1283 = node-c288() -> ()  [unwired: 2 out]
    n1284 = event shown="[0] \"Pane\": Mouse Down" {
      selector: _ -> [_ _]
      dyn-events: _ -> [_ _]
      timeout: _ -> [_ _]
      tunnel: w1973 -> [w1977 _]
      event Mouse Down {
        n1285 = event-data() -> ("Time"=w1979:u32, "Coords"=w1978:T8, "Button"=w1980:u16)  [unwired: 6 out]
        n1286 = case shown="1" w1980 {
          tunnel: w1979 -> [_ _ w2083]
          tunnel: w1978 -> [_ w2017 w2081]
          tunnel: w1977 -> [_ _ w2079]
          frame 0, Default {
          }
          frame 1 {
            n1287 = property on="APD 2" class="ImageControl"() -> ("Displayed Image Position"=w1987:cluster{"Left":i32, "Top":i32})  [unwired: 2 in, 2 out]
            n1288 = property on="APD 1" class="ImageControl"() -> ("Displayed Image Position"=w2016:cluster{"Left":i32, "Top":i32})  [unwired: 2 in, 2 out]
            n1289 = property on="Detection Laser X" class="ImageControl"() -> ("Displayed Image Position"=w2013:cluster{"Left":i32, "Top":i32})  [unwired: 2 in, 2 out]
            n1290 = property on="Detection Laser Y" class="ImageControl"() -> ("Displayed Image Position"=w2012:cluster{"Left":i32, "Top":i32})  [unwired: 2 in, 2 out]
            n1291 = property on="APD 2" class="ImageControl"() -> ("Displayed Image Size"=w1986:cluster{"Width":u32, "Height":u32})  [unwired: 2 in, 2 out]
            n1292 = property on="APD 1" class="ImageControl"() -> ("Displayed Image Size"=w2014:cluster{"Width":u32, "Height":u32})  [unwired: 2 in, 2 out]
            n1293 = property on="Detection Laser X" class="ImageControl"() -> ("Displayed Image Size"=w2015:cluster{"Width":u32, "Height":u32})  [unwired: 2 in, 2 out]
            n1294 = property on="Detection Laser Y" class="ImageControl"() -> ("Displayed Image Size"=w2011:cluster{"Width":u32, "Height":u32})  [unwired: 2 in, 2 out]
            n1295 = Unbundle By Name(w1986) -> ("Width"=w1983:u32, "Height"=w1982:u32)
            n1296 = Unbundle By Name(w1987) -> ("Left"=w1985:i32, "Top"=w1984:i32)
            n1297 = Unbundle By Name(w2014) -> ("Width"=w2008:u32, "Height"=w2007:u32)
            n1298 = Unbundle By Name(w2015) -> ("Width"=w2004:u32, "Height"=w2003:u32)
            n1299 = Unbundle By Name(w2011) -> ("Width"=w2000:u32, "Height"=w1999:u32)
            n1300 = Unbundle By Name(w2016) -> ("Left"=w2010:i32, "Top"=w2009:i32)
            n1301 = Unbundle By Name(w2013) -> ("Left"=w2006:i32, "Top"=w2005:i32)
            n1302 = Unbundle By Name(w2012) -> ("Left"=w2002:i32, "Top"=w2001:i32)
            n1303 = Bundle("Left"=w1985, "Top"=w1984, "Width"=w1983, "Height"=w1982) -> (w1981:T34)  [unwired: 1 in]
            n1304 = Bundle("Left"=w2010, "Top"=w2009, "Width"=w2008, "Height"=w2007) -> (w1998:T34)  [unwired: 1 in]
            n1305 = Bundle("Left"=w2006, "Top"=w2005, "Width"=w2004, "Height"=w2003) -> (w1997:T34)  [unwired: 1 in]
            n1306 = Bundle("Left"=w2002, "Top"=w2001, "Width"=w2000, "Height"=w1999) -> (w1996:T34)  [unwired: 1 in]
            n1307 = Build Cluster Array(w1981, w1998, w1997, w1996) -> (w1995:T35)
            n1308 = for {
              tunnel: w2017 -> [w2028]
              tunnel: w1995 -> [w2029] mode=indexing
              shift-right: [w2026] -> w1993
              shift-left: TRUE -> [w2027]
              shift-right: [w2025] -> w1991
              shift-left: _ -> [w2021]
              shift-right: [w2024] -> w1990
              shift-left: _ -> [w2020]
              shift-right: [w2023] -> w1989
              shift-left: _ -> [w2019]
              shift-right: [w2022] -> w1988
              shift-left: _ -> [w2018]
              n1309 = case shown="True" w2027 {
                selector: w2027 -> [w2034 _]
                tunnel: w2029 -> [_ w2043]
                tunnel: w2028 -> [_ w2041]
                tunnel: [w2034 w2039] -> w2026
                tunnel: [w2033 w2038] -> w2025
                tunnel: [w2032 w2037] -> w2024
                tunnel: [w2031 w2036] -> w2023
                tunnel: [w2030 w2035] -> w2022
                tunnel: w2021 -> [w2033 _]
                tunnel: w2020 -> [w2032 _]
                tunnel: w2019 -> [w2031 _]
                tunnel: w2018 -> [w2030 _]
                frame False {
                }
                frame True {
                  n1310 = Unbundle(w2043) -> (w2042:T34)
                  n1311 = call "isclickinwindow.vi"("Image Param"=w2042, "Point32"=w2041) -> ("4 Y"=w2035:i32, "3 Height"=w2036:i32, "2 X"=w2037:i32, "1 Width"=w2038:i32, "In image?"=w2040:bool)  [unwired: 1 in]
                  n1312 = Not(x=w2040) -> (.not. x?=w2039:bool)
                }
              }
            }
            n1313 = Not(x=w1993) -> (.not. x?=w1992:bool)
            n1314 = case shown="True" w1992 {
              tunnel: w1990 -> [_ w2056]
              tunnel: w1988 -> [_ w2055]
              tunnel: w1991 -> [_ w2054]
              tunnel: w1989 -> [_ w2053]
              frame False {
              }
              frame True {
                w2049 = FALSE ("Get Point")
                n1315 = local read "Scan lines (y)"() -> (w2058:u64)
                n1316 = local read "Actual MCL Inc (V)"() -> (w2050:dbl)
                n1317 = local read "Scan steps (MCL)"() -> (w2057:u64)
                n1318 = Divide "Y Pix/step"(x=w2053, y=w2058) -> (x/y=w2065:dbl)
                n1319 = Divide "Y V/pix"(x=w2050, y=w2065) -> (x/y=w2064:dbl)
                n1320 = Divide "Y half step offset"(x=w2050, y=2.0) -> (x/y=w2066:dbl)
                n1321 = Divide "X pix/step"(x=w2054, y=w2057) -> (x/y=w2063:dbl)
                n1322 = Negate(x=w2066) -> (-x=w2067:dbl)
                n1323 = local read "Initial Y"() -> (w2073:dbl)
                n1324 = Multiply(x=w2055, y=w2064) -> (x*y=w2074:dbl)
                n1325 = Divide "X half step offset"(x=w2050, y=2.0) -> (x/y=w2060:dbl)
                n1326 = Divide "X V/pix"(x=w2050, y=w2063) -> (x/y=w2062:dbl)
                n1327 = Multiply(x=w2050, y=w2057) -> (x*y=w2069:dbl)
                n1328 = Compound Arithmetic op=ADD(w2067, w2074, w2073) -> (w2051:dbl)
                "Pointer Y (V)" <- w2051
                n1329 = Multiply(x=w2062, y=w2056) -> (x*y=w2071:dbl)
                n1330 = Negate(x=w2060) -> (-x=w2059:dbl)
                n1331 = local read "Initial X"() -> (w2072:dbl)
                n1332 = Negate(x=w2071) -> (-x=w2070:dbl)
                n1333 = Compound Arithmetic op=ADD(w2059, w2069, w2072, w2070) -> (w2052:dbl)
                "Pointer X (V)" <- w2052
                n1334 = Or(x="Set X Only", y="Set Confocal Spot (X-Y)") -> (x .or. y?=w2045:bool)
                n1335 = Or(x="Set Confocal Spot (X-Y)", y="Set Y Only") -> (x .or. y?=w2044:bool)
                n1336 = case shown="True" w2045 {
                  tunnel: w2052 -> [_ w2075]
                  frame False {
                  }
                  frame True {
                    n1337 = property on="AO2" class="Slide (strict)"("Val(Sgnl)"=w2075) -> ()  [unwired: 2 in, 2 out]
                  }
                }
                n1338 = case shown="True" w2044 {
                  tunnel: w2051 -> [_ w2076]
                  frame False {
                  }
                  frame True {
                    n1339 = property on="AO1" class="Slide (strict)"("Val(Sgnl)"=w2076) -> ()  [unwired: 2 in, 2 out]
                  }
                }
                n1340 = local write "Set Confocal Spot (X-Y)"(w2049) -> ()
                n1341 = local write "Set X Only"(w2049) -> ()
                n1342 = local write "Set Y Only"(w2049) -> ()
              }
            }
          }
          frame 3 {
            n1343 = local read "BD 2 Frequency 1 (MHz)"() -> (w2077:dbl)
            n1344 = local read "BD 1 Frequency 1 (MHz)"() -> (w2078:dbl)
            n1345 = local write "Manipulating Trap"(TRUE ("Manipulating Trap")) -> ()
            n1346 = local write "Coords"(T8 {"Horizontal"=0, "Vertical"=0} ("Coords")) -> ()
            n1347 = while {
              tunnel: w2083 -> [w2088]
              tunnel: w2081 -> [w2087]
              tunnel: w2079 -> [w2086]
              tunnel: w2078 -> [w2085]
              tunnel: w2077 -> [w2084]
              stop <- w2089 stop-if-true
              n1348 = event shown="[0] \"Pane\": Mouse Move" {
                selector: _ -> [_ _]
                dyn-events: _ -> [_ _]
                timeout: _ -> [_ _]
                tunnel: ["Force Manip Abort" w2153] -> w2089
                tunnel: w2088 -> [w2096 _]
                tunnel: w2087 -> [w2094 _]
                tunnel: w2086 -> [w2093 _]
                tunnel: w2085 -> [w2092 _]
                tunnel: w2084 -> [w2091 _]
                event Mouse Move {
                  n1349 = event-data() -> ("Time"=w2097:u32, "Coords"=w2098:T8)  [unwired: 3 out]
                  n1350 = Less?(x=w2097, y=w2096) -> (x < y?=w2095:bool)
                  n1351 = case "Makes sure old motion events prior to mouse click aren't used" shown="False" w2095 {
                    tunnel: w2098 -> [w2140 _]
                    tunnel: w2094 -> [w2141 _]
                    tunnel: w2093 -> [w2118 _]
                    tunnel: w2092 -> [w2114 _]
                    tunnel: w2091 -> [w2113 _]
                    frame False {
                      n1352 = Subtract(x=w2140, y=w2141) -> (x-y=w2139:T8)
                      "Coords" <- w2139
                      n1353 = local read "Y RF Frequency Limits (MHz)"() -> (w2099:T17)
